vi "LUT - Test Get All.vi"(8 "error in (no error)":errorcluster) -> (0 "error out":errorcluster)   [LabVIEW 2017]
uses:
  <vilib>/addons/_JKI Toolkits/Caraya/classes/Assert/Assert True.vi
  <vilib>/addons/_JKI Toolkits/Caraya/classes/Assert/Assert Equal Value_Variant.vi
  <vilib>/addons/_JKI Toolkits/Caraya/classes/Assert/Assert Equal Value and Type_Variant.vi
  <vilib>/addons/_JKI Toolkits/Caraya/classes/Test/Test.lvclass
  src/LUT/LUT.lvclass
  <vilib>/addons/_JKI Toolkits/Caraya/classes/Assert/Assert.lvclass
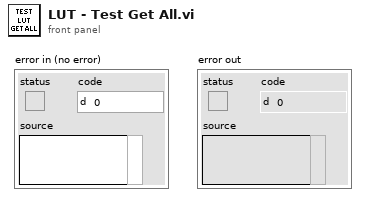
[diagram p1: front panel]
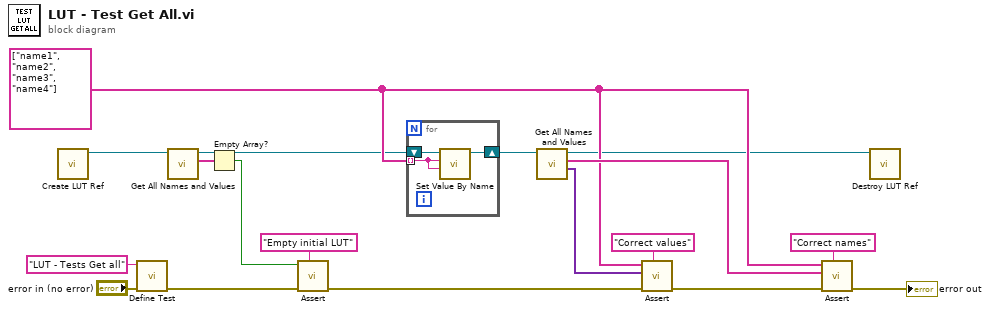
[diagram p0: block diagram]
diagram:
  w9 = string[] ["name1", "name2", "name3", "name4"]
  n1 = call "Create LUT Ref.vi"() -> ("LUT out"=w6:refnum<class "LUT.lvclass">)  [unwired: 10 in, 1 out]
  n2 = call <vilib>:"Define Test.vi"("error in (no error)"="error in (no error)", "Label (VI Title)"="LUT - Tests Get all") -> ("error out"=w3:errorcluster)  [unwired: 9 in]
  n3 = call "Get All Names and Values.vi"("LUT in"=w6) -> ("Names"=w7:string[], "LUT out"=w5:refnum<class "LUT.lvclass">)  [unwired: 7 in, 2 out]
  n4 = Empty Array?(array=w7) -> (empty?=w1:bool)
  n5 = call-poly <vilib>:"Assert.vi"("Label"="Empty initial LUT", "error in (no error)"=w3, "True?"=w1) -> ("error out"=w2:errorcluster)  [unwired: 8 in]
  n6 = for {
    shift-right: [w20] -> w16
    shift-left: w5 -> [w21]
    tunnel: w9 -> [w19] mode=indexing
    n7 = call "Set Value By Name.vi"("Value"=w19, "Name"=w19, "LUT in"=w21) -> ("LUT out"=w20:refnum<class "LUT.lvclass">)  [unwired: 6 in, 2 out]
  }
  n8 = call "Get All Names and Values.vi"("LUT in"=w16) -> ("Values"=w10:variant[], "Names"=w12:string[], "LUT out"=w8:refnum<class "LUT.lvclass">)  [unwired: 7 in, 1 out]
  n9 = call-poly <vilib>:"Assert.vi"("Label"="Correct values", "error in (no error)"=w2, "Y"=w10, "X"=w9) -> ("error out"=w14:errorcluster)  [unwired: 7 in]
  n10 = call-poly <vilib>:"Assert.vi"("Label"="Correct names", "error in (no error)"=w14, "Y"=w12, "X"=w9) -> ("error out"=→"error out":errorcluster)  [unwired: 7 in]
  n11 = call "Destroy LUT Ref.vi"("LUT in"=w8) -> ()  [unwired: 10 in, 1 out]
